vi "Test Open or Create 2.vi"(11 "Test Case In":refnum<class "Test Open Xml.lvclass">) -> (0 "error out":errorcluster, 3 "Test Case Out":refnum<class "Test Open Xml.lvclass">)   [LabVIEW 2020, in "Test Open Xml.lvclass"]
uses:
  Test Open Xml.lvclass
  Source/Open Xml.lvlib
  2c4bb252-386c-45a5-bd4c-bbe84a65a97e.vi
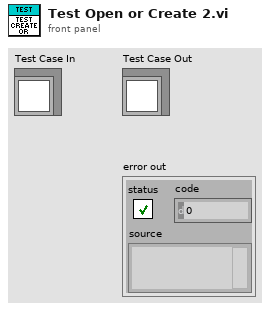
[diagram p1: front panel]
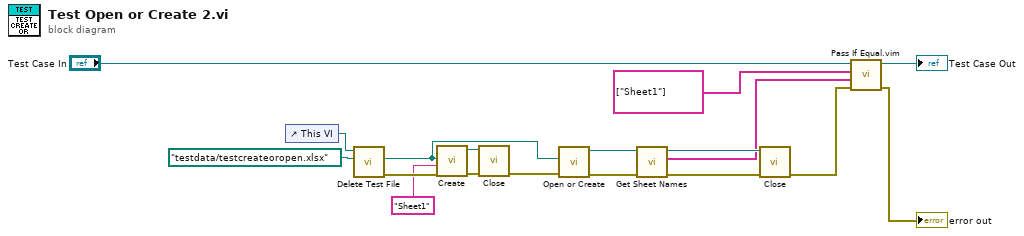
[diagram p0: block diagram]
diagram:
  n1 = control-ref of="This VI"() -> (w15:refnum<vi>)
  n2 = call "Delete Test File.vi"("name or relative path"=path "testdata/testcreateoropen.xlsx", "VI in"=w15) -> ("error out"=w11:errorcluster, "deleted path"=w9:path)  [unwired: 8 in]
  n3 = call "Create.vi"("error in"=w11, "SheetName"="Sheet1", "Path"=w9) -> ("error out"=w7:errorcluster, "SpreadsheetDoc"=w8:refnum<k24>)  [unwired: 7 in]
  n4 = call "Close.vi"("error in"=w7, "SpreadsheetDoc"=w8) -> ("error out"=w6:errorcluster)  [unwired: 9 in]
  n5 = call "Open or Create.vi"("error in"=w6, "Path"=w9) -> ("error out"=w12:errorcluster, "SpreadsheetDoc"=w4:refnum<k24>)  [unwired: 8 in]
  n6 = call "Get Sheet Names.vi"("error in"=w12, "SpreadsheetDoc in"=w4) -> ("error out"=w5:errorcluster, "Sheet Names"=w1:string[], "SpreadsheetDoc out"=w3:refnum<k24>)  [unwired: 7 in]
  n7 = call "Close.vi"("error in"=w5, "SpreadsheetDoc"=w3) -> ("error out"=w13:errorcluster)  [unwired: 9 in]
  n8 = call "Pass If Equal.vim"("error in (no error)"=w13, "Actual"=w1, "Expected"=string[] ["Sheet1"] ("Sheet Names"), "LUnit Test Case In"="Test Case In") -> ("error out"=→"error out":errorcluster, "LUnit Test Case Out"=→"Test Case Out":refnum<class "Test Open Xml.lvclass">)  [unwired: 6 in]
